vi "Interposer.vi"() -> ()   [LabVIEW 2013]
uses:
  Globals/Homes.vi
  <vilib>/Rock Robotics/WPI/Joystick/WPI_JoystickGetSetRefNum.vi
  Globals/Useful Values.vi
  <vilib>/addons/control/pid/pid.llb/PID (DBL).vi
  <vilib>/addons/control/pid/NI_PID_pid.lvlib
panel:
  out "Setpoint":dbl
  in  "PID gains":T1={"proportional gain (Kc)"=0.75, "integral time (Ti, min)"=0.0, "derivative time (Td, min)"=0.0} {"derivative time (Td, min)" format="%.3f"; "integral time (Ti, min)" format="%.3f"; "proportional gain (Kc)" format="%.3f"}
  out "Interposer Voltage":dbl
  out "Interposer Output":dbl
  in  "Negate?":bool
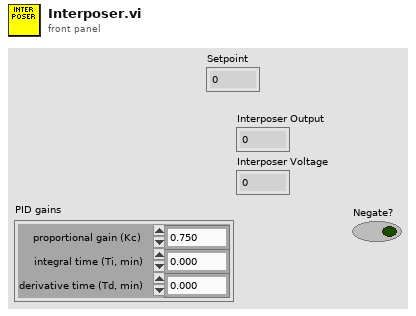
[diagram p1: front panel]
types:
  T1 = cluster{"proportional gain (Kc)":dbl, "integral time (Ti, min)":dbl, "derivative time (Td, min)":dbl}
  T2 = typedef "WPI_MotorControlDeviceRef.ctl" = cluster{"DeviceStatus":errorcluster, "Type":enum16{"PWM", "CAN"}, "PWM":cluster{"Digital Module":T3, "PWM Channel":T4, "DeadBand":T5}, "CAN":cluster{"Device Number":u8, "Control Mode":T6, "Semaphore":T7, "Max Vout":dbl}, "Invert":bool, "TransformRef":T8, "InvTransformRef":T8}
  T3 = typedef "FPGA_TypedefDigitalModule.ctl" = enum16{"Digital Module 1", "Digital Module 2"}
  T4 = typedef "FPGA_DIOPWMChannel.ctl" = enum8{"PWM 1", "PWM 2", "PWM 3", "PWM 4", "PWM 5", "PWM 6", "PWM 7", "PWM 8", "PWM 9", "PWM 10", "Invalid"}
  T5 = typedef "WPI_PWMDeadband.ctl" = cluster{"Name":string, "maxPositivePwm":i32, "minPositivePwm":i32, "centerPwm":i32, "maxNegativePwm":i32, "minNegativePwm":i32, "angularRange":u16}
  T6 = typedef "WPI_CANJaguar_ControlMode.ctl" = enum8{"Percent VBus", "Current", "Speed", "Position", "Voltage"}
  T7 = typedef "Semaphore RefNum" = refnum<k1>
  T8 = typedef "WPI_PWMTransform_ConPane.ctl" = refnum<vi>
  T9 = typedef "WPI_JoystickDevRef.ctl" = cluster{"Device":T10}
  T10 = typedef "WPI_JoystickDeviceEnum.ctl" = enum16{"USB 1", "USB 2", "USB 3", "USB 4", "Kinect 1", "Kinect 2"}
  T11 = typedef "WPI_AnalogChannelDevRef.ctl" = cluster{"DevStatus":errorcluster, "Analog Module":T12, "Analog Channel":T13}
  T12 = typedef "FPGA_TypedefAnalogModule.ctl" = enum16{"Analog Module 1", "Analog Module 2"}
  T13 = typedef "FPGA_AIChannel.ctl" = enum8{"AI 1", "AI 2", "AI 3", "AI 4", "AI 5", "AI 6", "AI 7", "AI 8", "Invalid"}
  T14 = typedef "WPI_JoystickButtonState.ctl" = cluster{"Button 1":bool, "Button 2":bool, "Button 3":bool, "Button 4":bool, "Button 5":bool, "Button 6":bool, "Button 7":bool, "Button 8":bool, "Button 9":bool, "Button 10":bool, "Button 11":bool, "Button 12":bool}
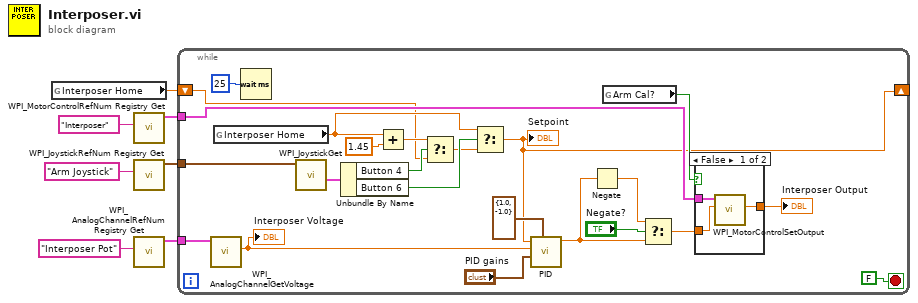
[diagram p0: block diagram]
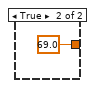
[diagram p2: hidden frame]
diagram:
  n1 = global read "Homes.vi" "Interposer Home"() -> (w1:dbl)
  n2 = call <vilib>:"WPI_MotorControlRefNum Registry Get.vi"("refnum name"="Interposer") -> ("MotorControlDevRef"=w4:T2)  [unwired: 9 in, 1 out]
  n3 = call <vilib>:"WPI_JoystickRefNum Registry Get.vi"("refnum name"="Arm Joystick") -> ("JoystickDevRef"=w6:T9)  [unwired: 9 in, 1 out]
  n4 = call <vilib>:"WPI_AnalogChannelRefNum Registry Get.vi"("refnum name"="Interposer Pot") -> ("AIDeviceRef"=w3:T11)  [unwired: 9 in, 1 out]
  n5 = while {
    tunnel: w6 -> [w29]
    tunnel: w4 -> [w17]
    tunnel: w3 -> [w25]
    shift-right: [w13] -> _
    shift-left: w1 -> [w9]
    stop <- FALSE stop-if-true
    n6 = call <vilib>:"WPI_AnalogChannelGetVoltage.vi"("AIDeviceRef"=w25) -> ("Voltage"=w26:dbl)  [unwired: 8 in, 2 out]
    "Interposer Voltage" <- w26
    n7 = global read "Homes.vi" "Interposer Home"() -> (w19:dbl)
    n8 = Wait (ms)(milliseconds to wait=u32 25) -> ()  [unwired: 1 out]
    n9 = call <vilib>:"WPI_JoystickGet.vi"("JoystickDevRef"=w29) -> ("Buttons"=w30:T14)  [unwired: 4 in, 2 out]
    n10 = Unbundle By Name(w30) -> ("Button 4"=w10:bool, "Button 6"=w12:bool)
    n11 = Add(x=w19, y=1.45) -> (x+y=w11:dbl)
    n12 = Select(t=w11, s=w10, f=w9) -> (s? t:f=w8:dbl)
    n13 = Select(t=w19, s=w12, f=w8) -> (s? t:f=w13:dbl)
    "Setpoint" <- w13
    n14 = call-poly <vilib>:"PID.vi"("output range"=cluster{"output high":dbl, "output low":dbl} {"output high"=1.0, "output low"=-1.0}, "PID gains"="PID gains", "process variable"=w26, "setpoint"=w13) -> ("output"=w23:dbl)  [unwired: 6 in, 1 out]
    n15 = Negate(x=w23) -> (-x=w24:dbl)
    n16 = global read "Useful Values.vi" "Arm Cal?"() -> (w18:bool)
    n17 = Select(t=w24, s="Negate?", f=w23) -> (s? t:f=w16:dbl)
    n18 = case shown="False" w18 {
      tunnel: w17 -> [w33 _]
      tunnel: w16 -> [w32 _]
      tunnel: [w31 69.0 ("Motor Output")] -> w15
      frame False {
        n19 = call <vilib>:"WPI_MotorControlSetOutput.vi"("Output"=w32, "MotorControlDevRef"=w33) -> ("Motor Output"=w31:dbl)  [unwired: 7 in, 2 out]
      }
      frame True {
      }
    }
    "Interposer Output" <- w15
  }
